vi "Table_Lookup_tl.vi"(4 "Lookup Table":string[][](table)=[["", "", "", ""], ["", "", "", ""], ["", "", "", ""]], 6 "Search String":string, 7 "Supplied variable":string, 8 "Required variable":string) -> (0 "Floating Output":dbl format="%.2f", 1 "Integer Output":i32, 2 "Outptut":string, 3 "Output row":string[](array[string]))   [LabVIEW 2010]
doc: "Looks down a named column of a headed table (default column 0) until search string is found, and outputs the value on the same row in the named column (default column 1). Also outputs the entire row on the matching line."
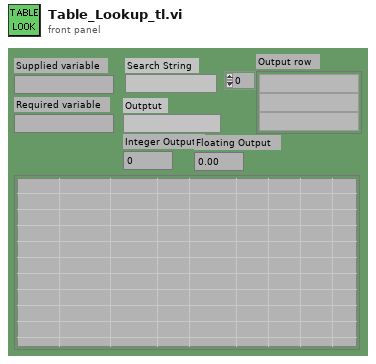
[diagram p1: front panel]
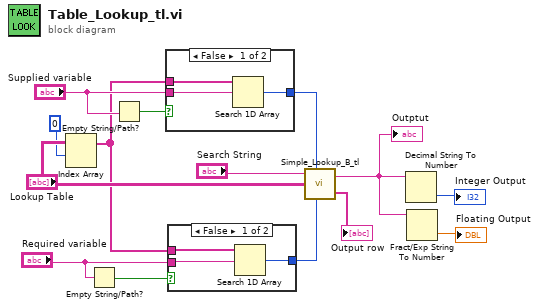
[diagram p0: block diagram]
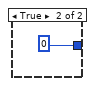
[diagram p2: hidden frame]
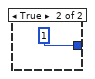
[diagram p3: hidden frame]
diagram:
  n1 = Index Array(array="Lookup Table", index (row)=0) -> (element=w5:string[])  [unwired: 1 in]
  n2 = Empty String/Path?(string/path="Required variable") -> (empty?=w13:bool)
  n3 = Empty String/Path?(string/path="Supplied variable") -> (empty?=w11:bool)
  n4 = case shown="False" w11 {
    tunnel: "Supplied variable" -> [w15 _]
    tunnel: [w17 0] -> w9
    tunnel: w5 -> [w16 _]
    frame False {
      n5 = Search 1D Array(1D array=w16, element=w15) -> (index of element=w17:i32)  [unwired: 1 in]
    }
    frame True {
    }
  }
  n6 = case shown="False" w13 {
    tunnel: "Required variable" -> [w19 _]
    tunnel: [w21 1] -> w12
    tunnel: w5 -> [w20 _]
    frame False {
      n7 = Search 1D Array(1D array=w20, element=w19) -> (index of element=w21:i32)  [unwired: 1 in]
    }
    frame True {
    }
  }
  n8 = call "Simple_Lookup_B_tl.vi"("Search String"="Search String", "Search Offset (0)"=w9, "Lookup Table"="Lookup Table", "Output Offset (1)"=w12) -> ("Output String"=w3:string, "Output row"=→"Output row":string[])  [unwired: 1 in]
  "Outptut" <- w3
  n9 = Decimal String To Number(string=w3) -> (number=→"Integer Output":i32)  [unwired: 2 in, 1 out]
  n10 = Fract/Exp String To Number(string=w3) -> (number=→"Floating Output":dbl)  [unwired: 3 in, 1 out]
